vi "Auto Probe Sense Value [PAS] Core.vi"(8 "error in (no error)":errorcluster, 10 "channel name (\"CHANNEL1\")":string="CHANNEL1", 11 "CS++Scope":refnum<class "CS++Scope.lvclass">) -> (0 "error out":errorcluster, 2 "auto probe sense value":dbl format="%.3f", 3 "CS++Scope out":refnum<class "CS++Scope.lvclass">)   [LabVIEW 2016, in "CS++Scope.lvlib" / "CS++Scope.lvclass"]
doc: "The VI returns the probe attenuation value the oscilloscope senses. You enable the automatic probe sense capability by setting the Probe Attenuation parameter of the IviScope Configure Channel VI to IVISCOPE_VAL_PROBE_SENSE_ON (-1).\n\nNote\n\n If you disable the automatic probe sense capability, this VI returns the manual probe attenuation setting."
uses:
  CS++Scope.lvclass
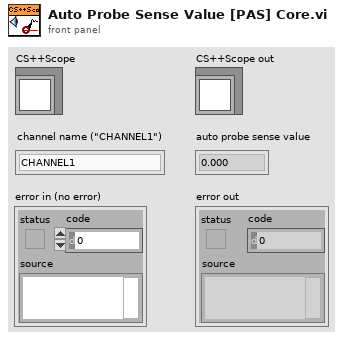
[diagram p1: front panel]
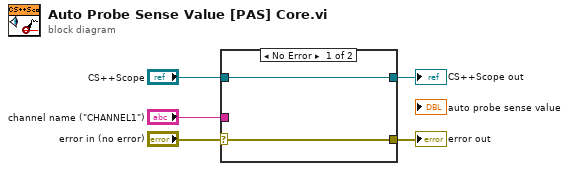
[diagram p0: block diagram]
diagram:
  n1 = case shown="No Error" "error in (no error)" {
    selector: "error in (no error)" -> [w6 w9]
    tunnel: [w6 w9] -> w4
    tunnel: [w7 w8] -> w2
    tunnel: "CS++Scope" -> [w7 w8]
    tunnel: "channel name (\"CHANNEL1\")" -> [_ _]
    frame No Error {
    }
    frame Error {
    }
  }
  "error out" <- w4
  "CS++Scope out" <- w2
